vi "Q2.vi"() -> ()   [LabVIEW 2014]
panel:
  out "Waveform Graph":i32[](graph)
  out "Array":dbl[](array[numeric])
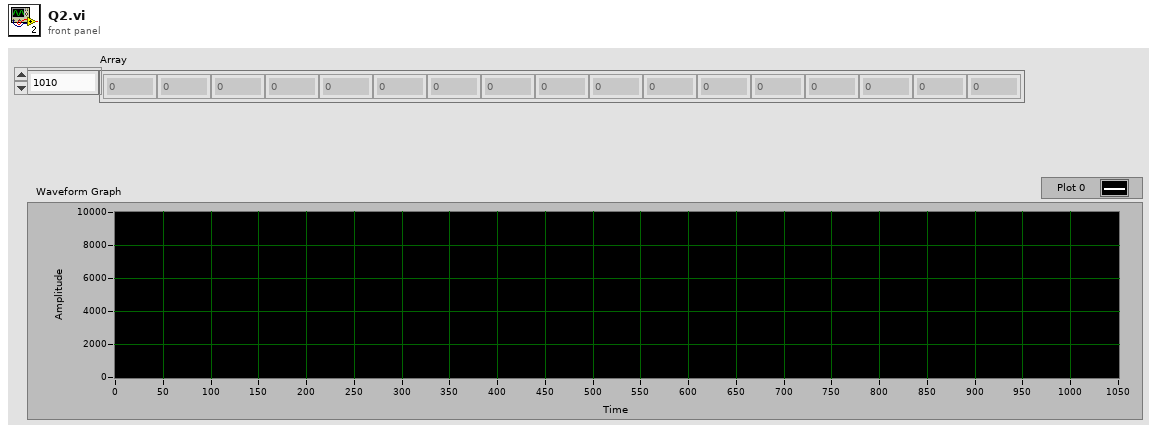
[diagram p1: front panel]
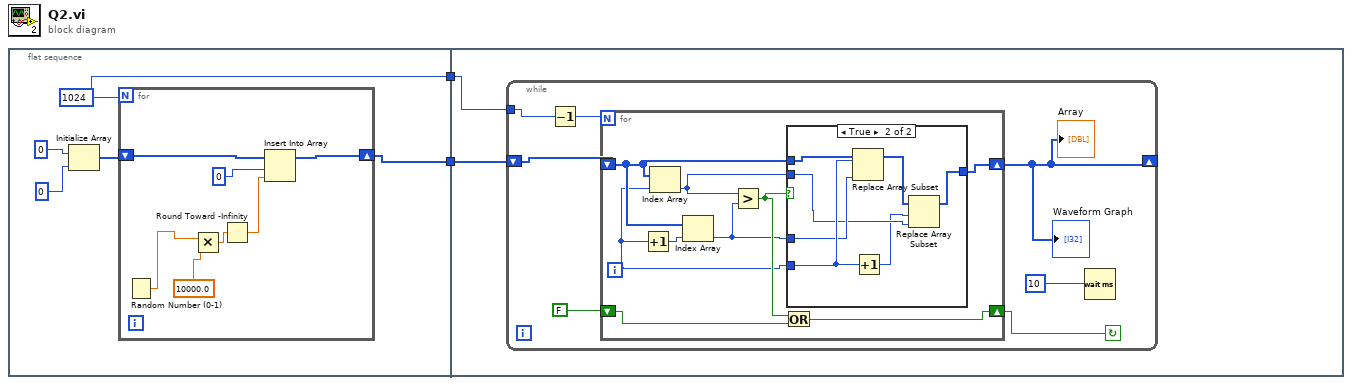
[diagram p0: block diagram]
diagram:
  n1 = flat-sequence {
    tunnel: [w4] -> w2
    tunnel: [w3] -> w1
    tunnel: w2 -> [w16]
    tunnel: w1 -> [w15]
    frame #0 {
      w3 = 1024
      n2 = Initialize Array(0, 0) -> (w7:i32[])
      n3 = for {
        N: w3 -> [_]
        shift-right: [w13] -> w4
        shift-left: w7 -> [w14]
        n4 = Random Number (0-1)() -> (number: 0 to 1=w12:dbl)
        n5 = Multiply(x=w12, y=10000.0) -> (x*y=w10:dbl)
        n6 = Round Toward -Infinity(1:w10) -> (0:w9:dbl)
        n7 = Insert Into Array(array=w14, index=0, new element=w9) -> (w13:i32[])
      }
    }
    frame #1 {
      n8 = while {
        shift-right: [w18] -> _
        shift-left: w16 -> [w23]
        tunnel: w15 -> [w19]
        stop <- w21 continue-if-true
        n9 = Decrement(x=w19) -> (x-1=w20:i32)
        n10 = for {
          N: w20 -> [_]
          shift-right: [w24] -> w18
          shift-left: w23 -> [w28]
          shift-right: [w31] -> w21
          shift-left: FALSE -> [w30]
          i -> [w27]
          n11 = Increment(x=w27) -> (x+1=w32:i32)
          n12 = Index Array(array=w28, index=w27) -> (element=w26:i32)
          n13 = Index Array(array=w28, index=w32) -> (element=w25:i32)
          n14 = Greater?(x=w26, y=w25) -> (0:w29:bool)
          n15 = Or(x=w29, y=w30) -> (x .or. y?=w31:bool)
          n16 = case shown="True" w29 {
            tunnel: w28 -> [w33 w40]
            tunnel: w27 -> [_ w39]
            tunnel: w26 -> [_ w36]
            tunnel: w25 -> [_ w38]
            tunnel: [w33 w34] -> w24
            frame False {
            }
            frame True {
              n17 = Replace Array Subset(array=w40, new element=w38, index=w39) -> (w37:i32[])
              n18 = Increment(x=w39) -> (x+1=w35:i32)
              n19 = Replace Array Subset(array=w37, new element=w36, index=w35) -> (w34:i32[])
            }
          }
        }
        "Array" <- w18
        "Waveform Graph" <- w18
        n20 = Wait (ms)(milliseconds to wait=10) -> ()  [unwired: 1 out]
      }
    }
  }
